vi "多设备同步_参考时钟同步.vi"() -> ()   [LabVIEW 2013]
uses:
  <userlib>/ArtDAQ/_SubVI/ArtDAQ_CreateAIVoltageChan.vi
  <userlib>/ArtDAQ/_SubVI/ArtDAQ_CfgSampClkTiming.vi
  <userlib>/ArtDAQ/_SubVI/ArtDAQ_CfgDigEdgeStartTrig.vi
  <userlib>/ArtDAQ/_SubVI/ArtDAQ_Read Analog DBL NChan NSamp.vi
panel:
  in  "通道1":string(combo)="Dev2/ai0"
  in  "通道0":string(combo)="Dev1/ai0"
  out "ErrorOutput":errorcluster caption="错误输出"
  out "?":dbl[][](graph)
  out "?":dbl[][](graph)
  in  "停止":bool
  # "备注: PCI设备可用RTSI_10M, PXIe设备可用PXIe_Clk100"
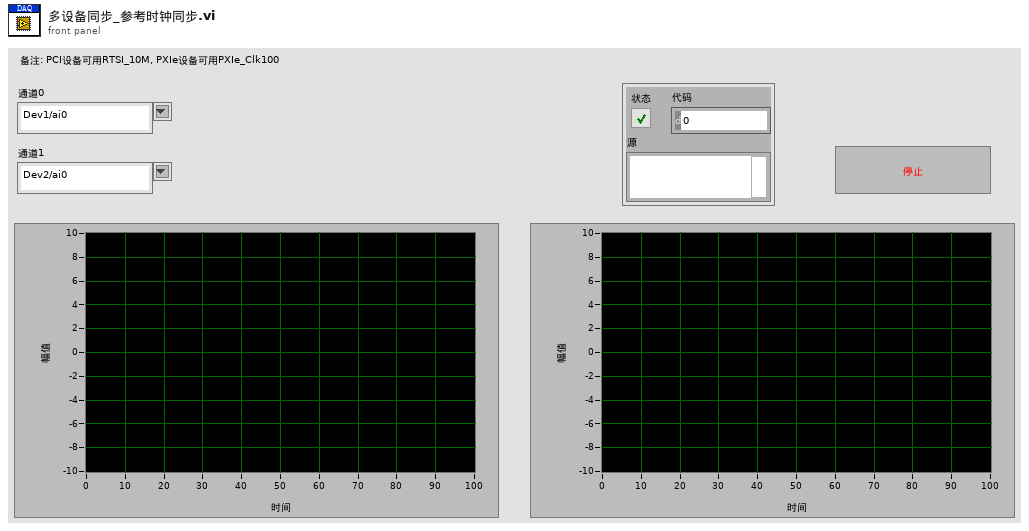
[diagram p1: front panel]
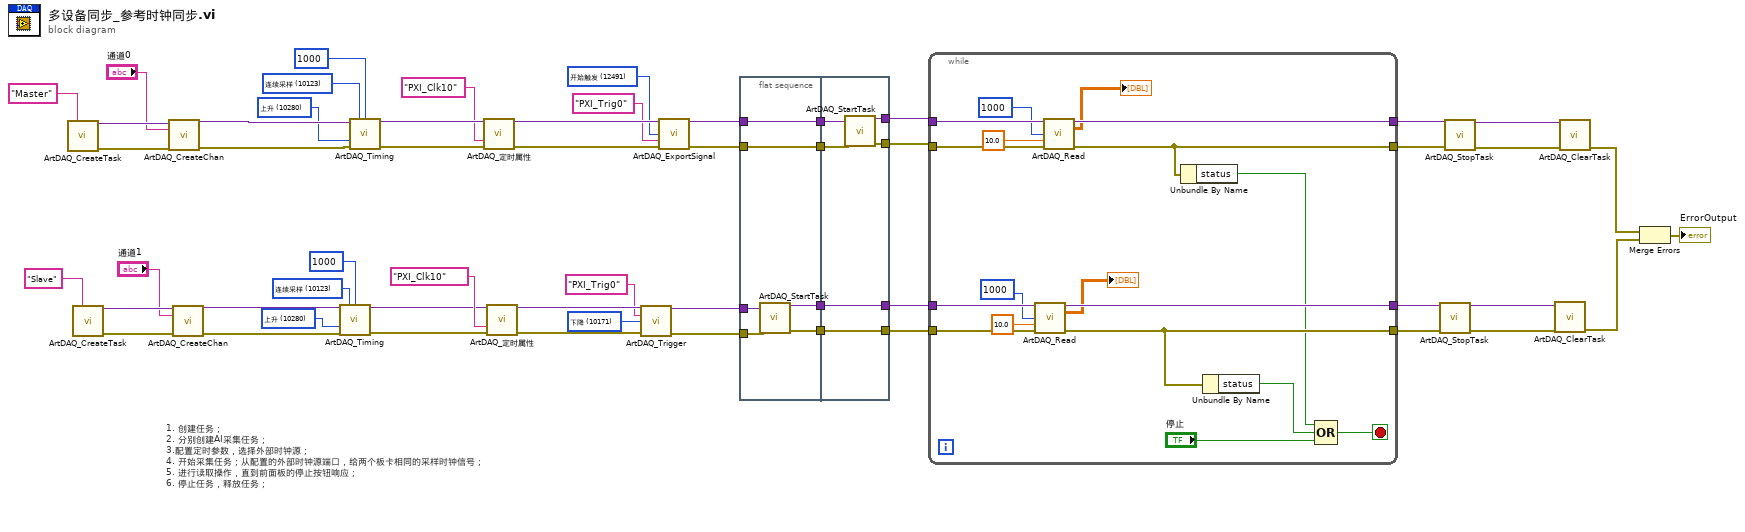
[diagram p0: block diagram]
diagram:
  w11 = 10171 items=["上升"=10280, "下降"=10171] ("边沿")
  w16 = 12491 items=["AI转换时钟"=12484, "10MHz参考时钟"=12535, "采样时钟"=12487, "开始触发"=12491, "暂停触发"=12489, "参考触发"=12490, "计数器输出事件"=12494, "主采样时钟时基"=12495, "同步脉冲输出"=12496, "位置比较事件"=10610, "检测更改事件"=12511, "频率输出"=12512] ("信号")
  w20 = 10280 items=["上升"=10280, "下降"=10171] ("边沿")
  w23 = 10280 items=["上升"=10280, "下降"=10171] ("边沿")
  w28 = 10123 items=["有限点采样"=10178, "连续采样"=10123] ("采样模式")
  w29 = 10123 items=["有限点采样"=10178, "连续采样"=10123] ("采样模式")
  # "1. 创建任务；\n2. 分别创建AI采集任务；\n3.配置定时参数，选择外部时钟源；\n4. 开始采集任务；从配置的外部时钟源端口，给两个板卡相同的采样时钟信号；\n5. 进行读取操作，直到前面板的停止按钮响应；\n6. 停止任务，释放任务；"
  n1 = call <userlib>:"ArtDAQ_CreateTask.vi"("任务名称"="Master" ("TaskName")) -> ("任务句柄"=w55:variant, "错误输出"=w54:errorcluster)  [unwired: 13 in]
  n2 = call <userlib>:"ArtDAQ_CreateTask.vi"("任务名称"="Slave" ("TaskName")) -> ("任务句柄"=w53:variant, "错误输出"=w52:errorcluster)  [unwired: 13 in]
  n3 = call-poly <userlib>:"ArtDAQ_CreateChan.vi"("任务句柄"=w55, "物理通道"="通道0", "错误输入"=w54) -> ("任务句柄"=w48:variant, "错误输出"=w49:errorcluster)  [unwired: 11 in]
  n4 = call-poly <userlib>:"ArtDAQ_CreateChan.vi"("任务句柄"=w53, "物理通道"="通道1", "错误输入"=w52) -> ("任务句柄"=w51:variant, "错误输出"=w50:errorcluster)  [unwired: 11 in]
  n5 = call-poly <userlib>:"ArtDAQ_Timing.vi"("任务句柄"=w51, "采样模式"=w28, "每通道采样数"=1000, "有效边沿"=w20, "错误输入"=w50) -> ("任务句柄"=w22:variant, "错误输出"=w21:errorcluster)  [unwired: 9 in]
  n6 = call-poly <userlib>:"ArtDAQ_Timing.vi"("任务句柄"=w48, "采样模式"=w29, "每通道采样数"=1000, "有效边沿"=w23, "错误输入"=w49) -> ("任务句柄"=w25:variant, "错误输出"=w24:errorcluster)  [unwired: 9 in]
  n7 = call-poly "ArtDAQ_定时属性.vi"("任务句柄"=w25, "参考时钟源"="PXI_Clk10", "错误输入"=w24) -> ("任务句柄"=w18:variant, "错误输出"=w17:errorcluster)  [unwired: 11 in]
  n8 = call-poly "ArtDAQ_定时属性.vi"("任务句柄"=w22, "参考时钟源"="PXI_Clk10" ("时钟源1"), "错误输入"=w21) -> ("任务句柄"=w14:variant, "错误输出"=w13:errorcluster)  [unwired: 11 in]
  n9 = call-poly <userlib>:"ArtDAQ_Trigger.vi"("任务句柄"=w14, "触发源"="PXI_Trig0" ("输出接线端"), "边沿"=w11, "错误输入"=w13) -> ("任务句柄"=w10:variant, "错误输出"=w9:errorcluster)  [unwired: 10 in]
  n10 = call <userlib>:"ArtDAQ_ExportSignal.vi"("任务句柄"=w18, "信号"=w16, "输出接线端"="PXI_Trig0", "错误输入"=w17) -> ("任务句柄"=w8:variant, "错误输出"=w7:errorcluster)  [unwired: 10 in]
  n11 = flat-sequence {
    tunnel: w10 -> [w59]
    tunnel: w9 -> [w58]
    tunnel: w8 -> [w57]
    tunnel: w7 -> [w56]
    tunnel: [w61] -> w6
    tunnel: [w60] -> w5
    tunnel: [w57] -> w4
    tunnel: [w56] -> w3
    tunnel: [w66] -> w46
    tunnel: [w67] -> w47
    tunnel: w6 -> [w67]
    tunnel: w5 -> [w66]
    tunnel: w4 -> [w65]
    tunnel: w3 -> [w64]
    tunnel: [w63] -> w2
    tunnel: [w62] -> w1
    frame #0 {
      n12 = call <userlib>:"ArtDAQ_StartTask.vi"("任务句柄"=w59, "错误输入"=w58) -> ("任务句柄"=w61:variant, "错误输出"=w60:errorcluster)  [unwired: 12 in]
    }
    frame #1 {
      n13 = call <userlib>:"ArtDAQ_StartTask.vi"("任务句柄"=w65, "错误输入"=w64) -> ("任务句柄"=w63:variant, "错误输出"=w62:errorcluster)  [unwired: 12 in]
    }
  }
  n14 = while {
    tunnel: w2 -> [w85]
    tunnel: w1 -> [w84]
    tunnel: w47 -> [w83]
    tunnel: w46 -> [w82]
    tunnel: [w81] -> w43
    tunnel: [w72] -> w42
    tunnel: [w80] -> w39
    tunnel: [w71] -> w38
    stop <- w77 stop-if-true
    n15 = call-poly <userlib>:"ArtDAQ_Read.vi"("任务句柄"=w83, "每通道采样数"=1000 ("NumSampsPerChan"), "超时s"=10.0 ("Timeout"), "错误输入"=w82) -> ("任务句柄"=w80:variant, "数据"=→"?":dbl[][], "错误输出"=w71:errorcluster)  [unwired: 8 in, 1 out]
    n16 = call-poly <userlib>:"ArtDAQ_Read.vi"("任务句柄"=w85, "每通道采样数"=1000 ("NumSampsPerChan"), "超时s"=10.0 ("Timeout"), "错误输入"=w84) -> ("任务句柄"=w81:variant, "数据"=→"?":dbl[][], "错误输出"=w72:errorcluster)  [unwired: 8 in, 1 out]
    n17 = Unbundle By Name(w72) -> ("status"=w70:bool)
    n18 = Unbundle By Name(w71) -> ("status"=w79:bool)
    n19 = Compound Arithmetic op=OR(w70, w79, "停止") -> (w77:bool)
  }
  n20 = call <userlib>:"ArtDAQ_StopTask.vi"("任务句柄"=w39, "错误输入"=w38) -> ("任务句柄"=w40:variant, "错误输出"=w41:errorcluster)  [unwired: 12 in]
  n21 = call <userlib>:"ArtDAQ_StopTask.vi"("任务句柄"=w43, "错误输入"=w42) -> ("任务句柄"=w45:variant, "错误输出"=w44:errorcluster)  [unwired: 12 in]
  n22 = call <userlib>:"ArtDAQ_ClearTask.vi"("任务句柄"=w40, "错误输入"=w41) -> ("错误输出"=w36:errorcluster)  [unwired: 13 in]
  n23 = call <userlib>:"ArtDAQ_ClearTask.vi"("任务句柄"=w45, "错误输入"=w44) -> ("错误输出"=w37:errorcluster)  [unwired: 13 in]
  n24 = Merge Errors(w37, w36) -> (→"ErrorOutput":errorcluster)
